vi "NUSP2RCRL.vi"(8 "error in":errorcluster, 10 "Número USP":dbl=4112767.0 format="%#_13g", 11 "Exercise Number":u32=1) -> (0 "error out":errorcluster, 3 "RC/RL Sim Param":T1={"V"=8.0, "C"=8.0, "R"=8.0, "L"=8.0, "RC/RL"=FALSE, "F"=8.0, "DCycle"=8.0})   [LabVIEW 2014]
uses:
  Ctls/RCSim Controls.ctl
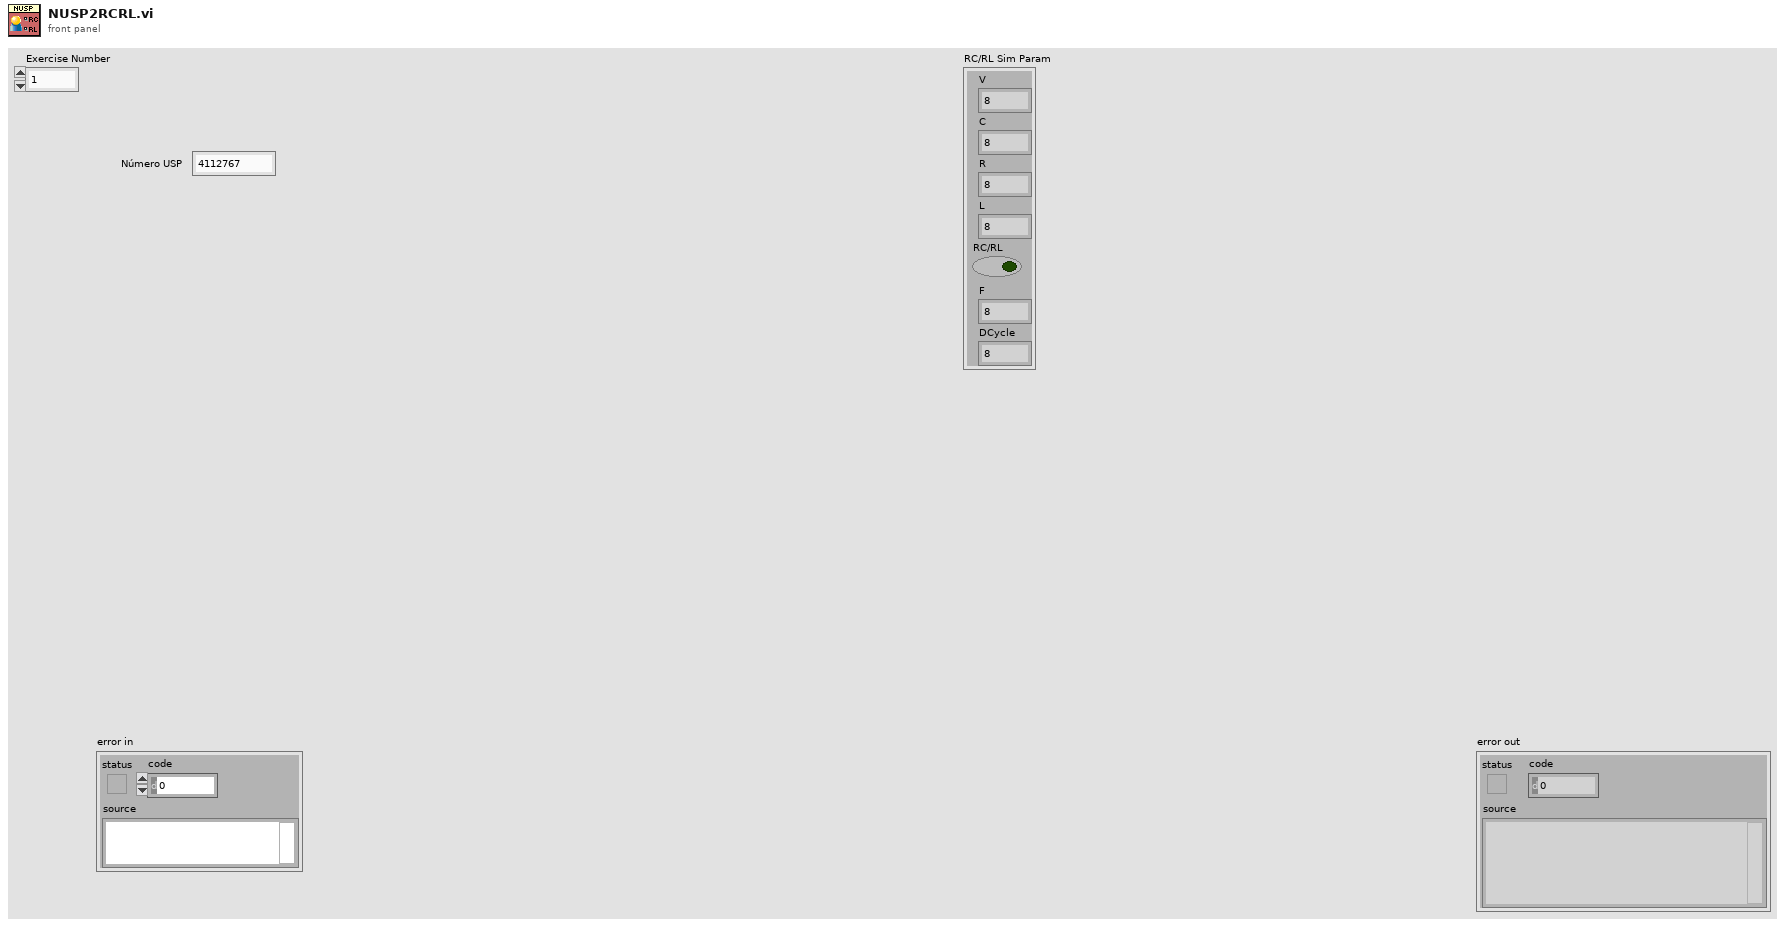
[diagram p1: front panel]
types:
  T1 = typedef "RCSim Controls.ctl" = cluster{"V":dbl, "C":dbl, "R":dbl, "L":dbl, "RC/RL":bool, "F":dbl, "DCycle":dbl}
  T2 = cluster{"standard deviation":dbl, "F1delta":dbl, "F2delta":dbl, "F3delta":dbl, "A1delta":dbl, "A2delta":dbl, "A3delta":dbl, "A3min":dbl, "A2min":dbl, "A1min":dbl, "F3min":dbl, "F2min":dbl, "F1min":dbl}
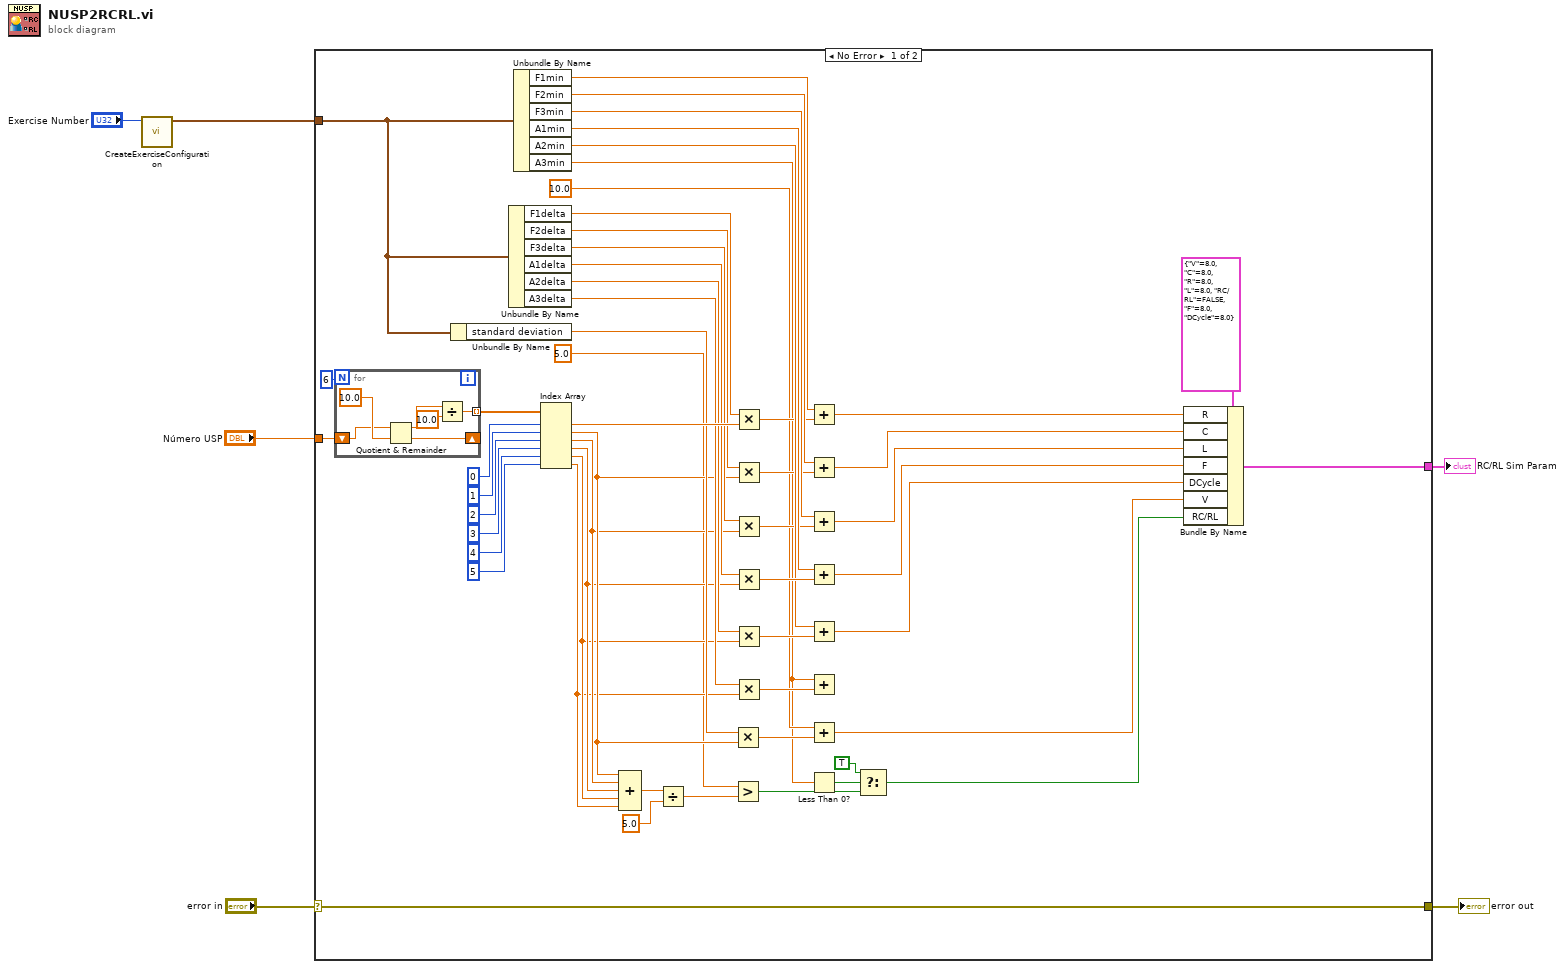
[diagram p0: block diagram]
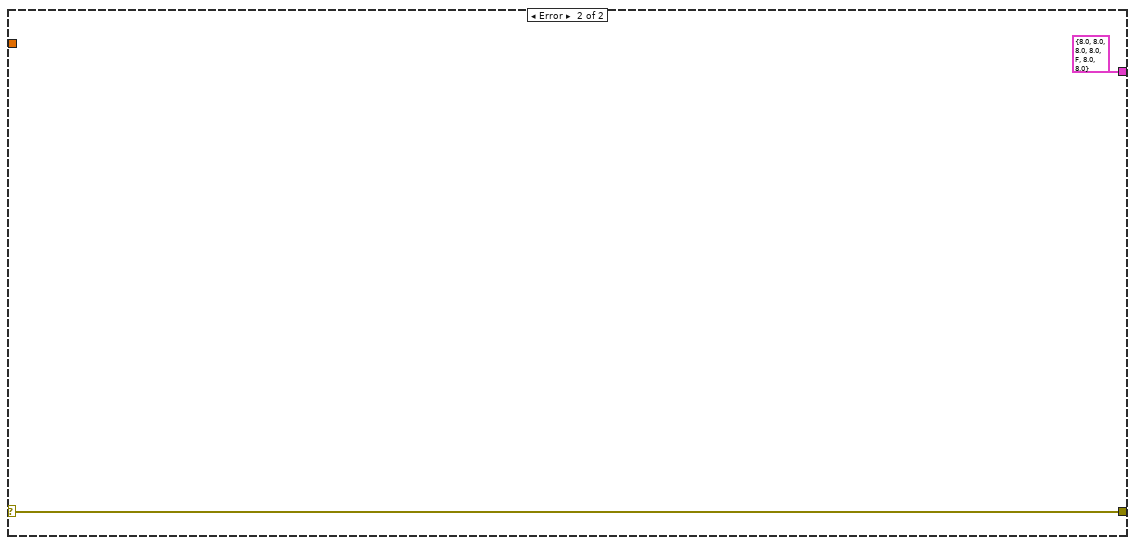
[diagram p2: hidden frame]
diagram:
  n1 = call "CreateExerciseConfiguration.vi"("Exercise Number"="Exercise Number") -> ("Exercise Configuration"=w1:T2)  [unwired: 9 in, 1 out]
  n2 = case shown="No Error" "error in" {
    selector: "error in" -> [w15 w68]
    tunnel: "Número USP" -> [w57 _]
    tunnel: [w15 w68] -> w4
    tunnel: w1 -> [w47 _]
    tunnel: [w16 T1 {"V"=8.0, "C"=8.0, "R"=8.0, "L"=8.0, "RC/RL"=FALSE, "F"=8.0, "DCycle"=8.0}] -> w3
    frame No Error {
      n3 = for {
        N: 6 -> [_]
        tunnel: [w61] -> w55 mode=indexing
        shift-right: [w64] -> _
        shift-left: w57 -> [w65]
        n4 = Quotient & Remainder(x=w65, y=10.0) -> (x-y*floor(x/y)=w63:dbl, floor(x/y)=w64:dbl)
        n5 = Divide(x=w63, y=10.0) -> (x/y=w61:dbl)
      }
      n6 = Unbundle By Name(w47) -> ("standard deviation"=w32:dbl)
      n7 = Unbundle By Name(w47) -> ("F1delta"=w46:dbl, "F2delta"=w45:dbl, "F3delta"=w44:dbl, "A1delta"=w43:dbl, "A2delta"=w42:dbl, "A3delta"=w41:dbl)
      n8 = Unbundle By Name(w47) -> ("F1min"=w40:dbl, "F2min"=w39:dbl, "F3min"=w38:dbl, "A1min"=w37:dbl, "A2min"=w36:dbl, "A3min"=w11:dbl)
      n9 = Index Array(array=w55, index #1=0 ("index"), index #2=1 ("index"), index #3=2 ("index"), index #4=3 ("index"), index #5=4 ("index"), index #6=5 ("index")) -> (element #1=w54:dbl, element #2=w29:dbl, element #3=w28:dbl, element #4=w27:dbl, element #5=w26:dbl, element #6=w25:dbl)
      n10 = Compound Arithmetic op=ADD(w29, w28, w27, w26, w25) -> (w22:dbl)
      n11 = Divide(x=w22, y=5.0) -> (x/y=w20:dbl)
      n12 = Multiply(x=w32, y=w29) -> (x*y=w31:dbl)
      n13 = Greater?(x=5.0 ("y"), y=w20) -> (0:w8:bool)
      n14 = Multiply(x=w46, y=w54) -> (x*y=w33:dbl)
      n15 = Multiply(x=w45, y=w29) -> (x*y=w34:dbl)
      n16 = Multiply(x=w44, y=w28) -> (x*y=w35:dbl)
      n17 = Multiply(x=w43, y=w27) -> (x*y=w60:dbl)
      n18 = Multiply(x=w42, y=w26) -> (x*y=w59:dbl)
      n19 = Multiply(x=w41, y=w25) -> (x*y=w58:dbl)
      n20 = Add(x=w40, y=w33) -> (x+y=w19:dbl)
      n21 = Add(x=w39, y=w34) -> (x+y=w18:dbl)
      n22 = Add(x=w38, y=w35) -> (x+y=w17:dbl)
      n23 = Add(x=w37, y=w60) -> (x+y=w13:dbl)
      n24 = Add(x=w36, y=w59) -> (x+y=w12:dbl)
      n25 = Add(x=w11, y=w58) -> ()  [unwired: 1 out]
      n26 = Add(x=10.0 ("y"), y=w31) -> (x+y=w14:dbl)
      n27 = Less Than 0?(x=w11) -> (x < 0?=w10:bool)
      n28 = Select(t=TRUE, s=w10, f=w8) -> (s? t:f=w7:bool)
      n29 = Bundle By Name(cluster=T1 {"V"=8.0, "C"=8.0, "R"=8.0, "L"=8.0, "RC/RL"=FALSE, "F"=8.0, "DCycle"=8.0}, "R"=w19, "C"=w18, "L"=w17, "F"=w13, "DCycle"=w12, "V"=w14, "RC/RL"=w7) -> (w16:T1)
    }
    frame Error {
    }
  }
  "error out" <- w4
  "RC/RL Sim Param" <- w3
